vi "ActTurn.vi"(9 "FirstTime":bool, 10 "MaxSpeed (ft/s)":dbl, 11 "Degrees":dbl) -> (0 "RotationSpeedDemand":dbl, 3 "Done":bool)   [LabVIEW 2020]
doc: "Robot will turn a set number of degrees utilizing position control \n\nInputs:\n-- MaxSpeed -- Double -- In ft/s, the MaxSpeed the robot can go -- \n-- Degrees -- Double -- Rotation in degrees you want the robot to go -- \n-- FirstTime -- Boolean -- Input true the first time this function is called, sets the target position -- \n\nOutputs:\n-- Done -- Bool -- has the robot reached its target distance -- \n-- LeftSpeedDemand -- Double -- Speed Demand for left drive train inorder to reach target -- \n-- RightSpeedDemand -- Double -- Speed Demand for left drive train inorder to reach target --"
uses:
  <vilib>/Rock Robotics/Network Tables/NT Write Number.vi
  <vilib>/Rock Robotics/Network Tables/NT Write Boolean.vi
  <vilib>/Rock Robotics/WPI/ThirdParty/JAS_Junk/TrajLib/Trajectory_Library.lvlib
panel:
  out "Unfiltetred Done":bool
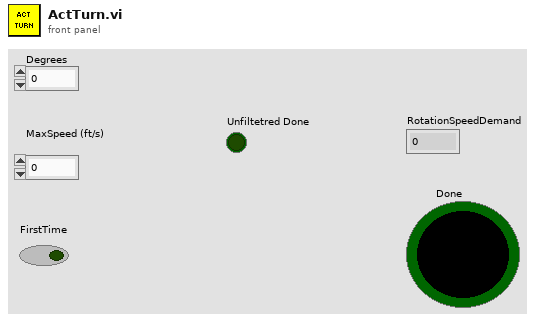
[diagram p1: front panel]
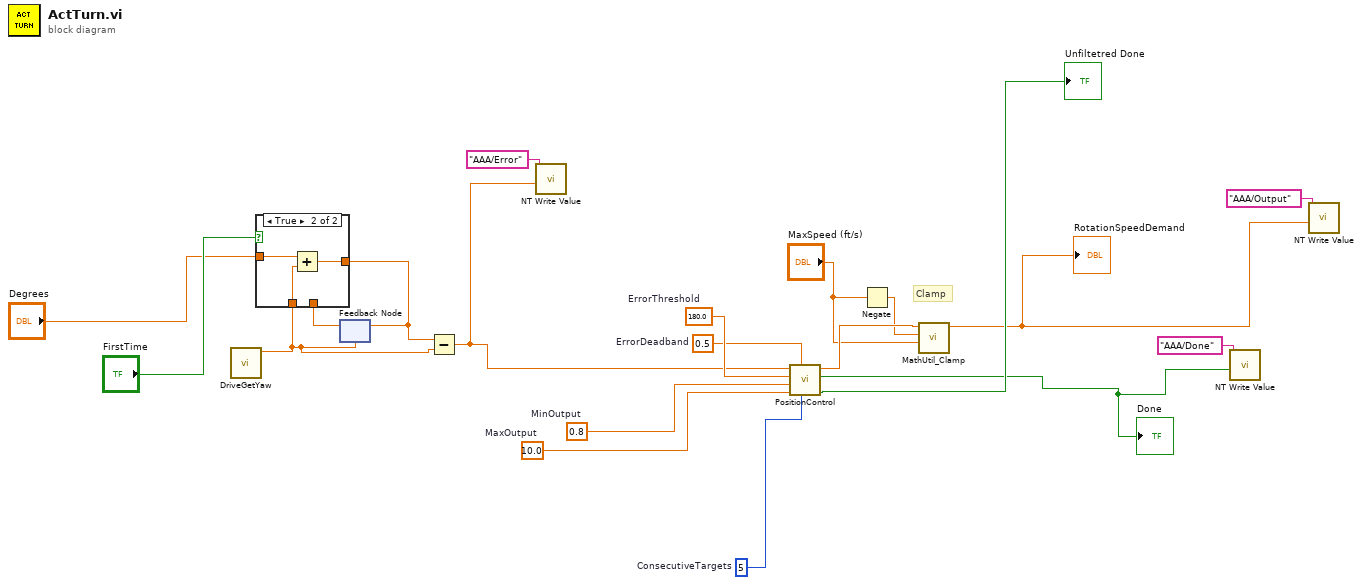
[diagram p0: block diagram]
diagram:
  w9 = 10.0  # MaxOutput
  w10 = 0.8  # MinOutput
  w15 = 5  # ConsecutiveTargets
  w16 = 0.5  # ErrorDeadband
  w17 = 180.0  # ErrorThreshold
  # "Clamp"
  n1 = call "DriveGetYaw.vi"() -> ("Yaw"=w7:dbl)  [unwired: 11 in]
  n2 = feedback #1(w7) -> (w18:dbl)
  n3 = case shown="True" "FirstTime" {
    tunnel: "Degrees" -> [_ w24]
    tunnel: [w21 w23] -> w11
    tunnel: w18 -> [w21 _]
    tunnel: w7 -> [_ w22]
    frame False {
    }
    frame True {
      n4 = Add(x=w24, y=w22) -> (x+y=w23:dbl)
    }
  }
  n5 = feedback-in #1(w11) -> ()
  n6 = Subtract(x=w11, y=w7) -> (x-y=w5:dbl)
  n7 = call-poly <vilib>:"NT Write Value.vi"("value"=w5, "name"="AAA/Error") -> ()  [unwired: 9 in, 1 out]
  n8 = call "PositionControl.vi"("ConsecutiveTargets"=w15, "ErrorDeadband"=w16, "MaxOutput"=w9, "MinOutput"=w10, "ErrorThreshold"=w17, "Error"=w5) -> ("UnfilteredOnTarget"=→"Unfiltetred Done":bool, "OnTarget"=w3:bool, "OutputValue"=w14:dbl)  [unwired: 3 in]
  "Done" <- w3
  n9 = Negate(x="MaxSpeed (ft/s)") -> (-x=w13:dbl)
  n10 = call <vilib>:"MathUtil_Clamp.vi"("High Limit"="MaxSpeed (ft/s)", "Low Limit"=w13, "Value"=w14) -> ("Result"=w1:dbl)  [unwired: 8 in]
  "RotationSpeedDemand" <- w1
  n11 = call-poly <vilib>:"NT Write Value.vi"("value"=w3, "name"="AAA/Done") -> ()  [unwired: 9 in, 1 out]
  n12 = call-poly <vilib>:"NT Write Value.vi"("value"=w1, "name"="AAA/Output") -> ()  [unwired: 9 in, 1 out]
